vi "Set_MultiVar_BulkMode_Value.vi"(8 "error in (no error)":errorcluster, 9 "varValue":dbl[](array[numeric]) format="%#_13g", 10 "varName":string, 11 "muExpr in":refnum<class "mupExpr.lvclass">) -> (0 "error out":errorcluster, 3 "muExpr out":refnum<class "mupExpr.lvclass">)   [LabVIEW 2015, in "mupExpr.lvclass"]
doc: "Set the bulk mode values for a selected variable.\n\nIf the variable is not found, a warning is generated."
uses:
  mupExpr.lvclass
  mupExpr.lvclass/mupExpr.ctl
  mupLib/mupSetVarValue_Array.vi
  <vilib>/Utility/error.llb/Error Cluster From Error Code.vi
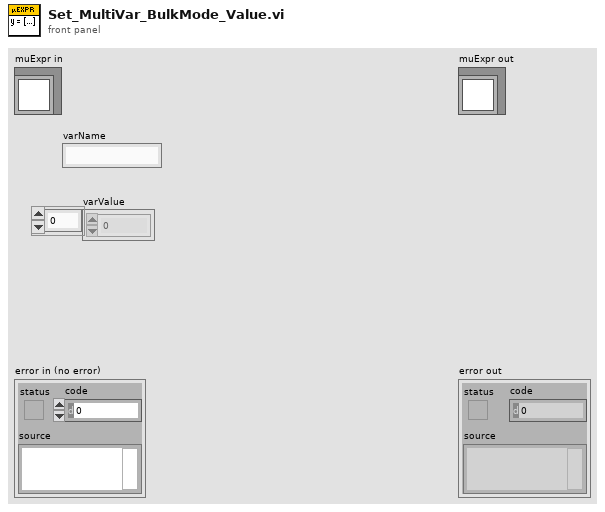
[diagram p1: front panel]
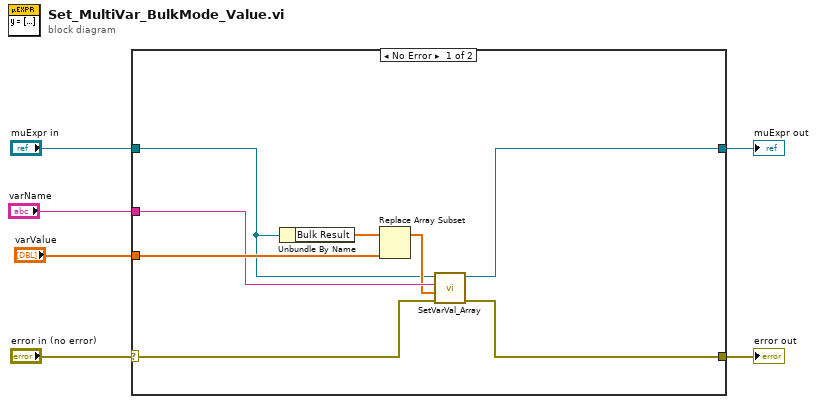
[diagram p0: block diagram]
diagram:
  n1 = case shown="No Error" "error in (no error)" {
    selector: "error in (no error)" -> [w8 w15]
    tunnel: "varValue" -> [w14 _]
    tunnel: "varName" -> [w13 _]
    tunnel: "muExpr in" -> [w10 w16]
    tunnel: [w7 w15] -> w3
    tunnel: [w9 w16] -> w2
    frame No Error {
      n2 = Unbundle By Name(w10) -> ("Bulk Result"=w12:dbl[])
      n3 = Replace Array Subset(array=w12, new element=w14) -> (w11:dbl[])  [unwired: 1 in]
      n4 = call "SetVarVal_Array.vi"("error in (no error)"=w8, "varValue"=w11, "varName"=w13, "muExpr in"=w10) -> ("error out"=w7:errorcluster, "muExpr out"=w9:refnum<class "mupExpr.lvclass">)  [unwired: 6 in]
    }
    frame Error {
    }
  }
  "error out" <- w3
  "muExpr out" <- w2
